vi "Test.vi"() -> ()   [LabVIEW 2019, in "ByteGSWebAPI.lvlib"]
uses:
  ByteGSWebAPI.lvlib
  BookingInstrument/Cntrls/PostBooking.ctl
  BookingInstrument/Cntrls/SingleBookingInstruments.ctl
  ByteGSWebAPI-V0.lvclass
panel:
  out "BookingList":T1[](array[typedef])
  in  "BookingInstrument":T2
  out "error out":errorcluster
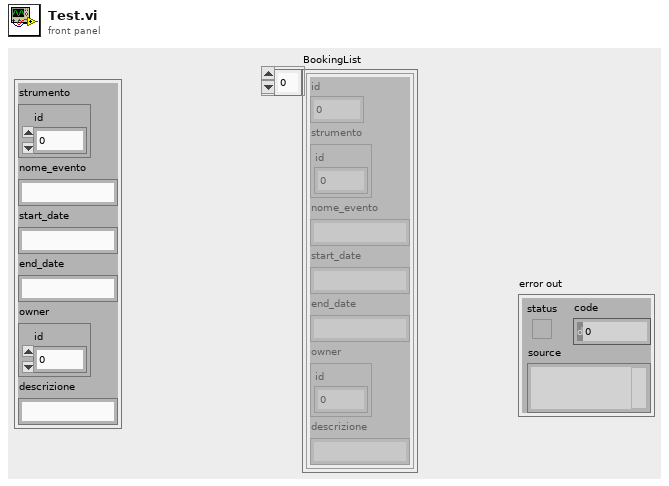
[diagram p1: front panel]
types:
  T1 = typedef "ByteGSWebAPI.lvlib/ByteGSWebAPI-V0.lvclass/SingleBookingInstruments.ctl" = cluster{"id":i32, "strumento":cluster{"id":i32}, "nome_evento":string, "start_date":string, "end_date":string, "owner":cluster{"id":i32}, "descrizione":string}
  T2 = typedef "ByteGSWebAPI.lvlib/ByteGSWebAPI-V0.lvclass/PostBooking.ctl" = cluster{"strumento":cluster{"id":i32}, "nome_evento":string, "start_date":string, "end_date":string, "owner":cluster{"id":i32}, "descrizione":string}
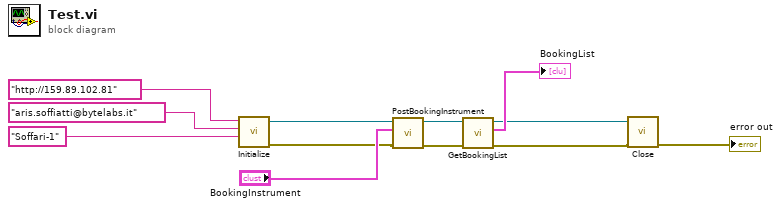
[diagram p0: block diagram]
diagram:
  n1 = call "Initialize.vi"("Password"="Soffari-1", "Username"="aris.soffiatti@bytelabs.it", "Server-URL"="http://159.89.102.81") -> ("error out"=w6:errorcluster, "ByteGSWebAPI-V0 out"=w8:refnum<class "ByteGSWebAPI-V0.lvclass">)  [unwired: 7 in]
  n2 = call-dynamic "PostBookingInstrument.vi"("error in (no error)"=w6, "BookingInstrument"="BookingInstrument", "ByteGSWebAPI-V0 in"=w8) -> ("error out"=w4:errorcluster, "ByteGSWebAPI-V0 out"=w5:refnum<class "ByteGSWebAPI-V0.lvclass">)  [unwired: 7 in]
  n3 = call-dynamic "GetBookingList.vi"("error in (no error)"=w4, "ByteGSWebAPI-V0 in"=w5) -> ("error out"=w1:errorcluster, "BookingList"=→"BookingList":T1[], "ByteGSWebAPI-V0 out"=w2:refnum<class "ByteGSWebAPI-V0.lvclass">)  [unwired: 7 in]
  n4 = call-dynamic "Close.vi"("error in (no error)"=w1, "ByteGSWebAPI-V0 in"=w2) -> ("error out"=→"error out":errorcluster)  [unwired: 8 in, 1 out]
